vi "Print.vi"(8 "error in":errorcluster, 11 "Object Type Base in":refnum<class "Object Type Base.lvclass">) -> (0 "error out":errorcluster, 2 "Fields":map{string, string}(c390), 3 "Object Type Base out":refnum<class "Object Type Base.lvclass">)   [LabVIEW 2024, in "EDS.lvlib" / "Object Type Base.lvclass"]
uses:
  Object Type Base.lvclass
  Object Type.ctl
  Data Type.ctl
  Access Type.ctl
  Object Type Base.lvclass/Object Type Base.ctl
  EDS.lvlib
panel:
  out "AccessType":T1=enum."const"
  out "DataType":T2 items=["BOOLEAN"=1, "INTEGER8"=2, "INTEGER16"=3, "INTEGER32"=4, "UNSIGNED8"=5, "UNSIGNED16"=6, "UNSIGNED32"=7, "REAL32"=8, "VISIBLE_STRING"=9, "OCTET_STRING"=10, "UNICODE_STRING"=11, "TIME_OF_DAY"=12, "TIME_DIFFERENCE"=13, "RESERVED1"=14, "DOMAIN"=15, "INTEGER24"=16, "REAL64"=17, "INTEGER40"=18, "INTEGER48"=19, "INTEGER56"=20, "INTEGER64"=21, "UNSIGNED24"=22, "RESERVED2"=23, "UNSIGNED40"=24, "UNSIGNED48"=25, "UNSIGNED56"=26, "UNSIGNED64"=27, "RESERVED3"=28, "RESERVED4"=29, "RESERVED5"=30, "RESERVED6"=31, "PDO_COMMUNICATION_PARAMETER"=32, "PDO_MAPPING"=33, "SDO_PARAMETER"=34, "IDENTITY"=35, "RESERVED7"=36]
  out "ObjectType":T3 items=["NULL"=0, "DOMAIN"=2, "DEFTYPE"=5, "DEFSTRUCT"=6, "VAR"=7, "ARRAY"=8, "RECORD"=9]
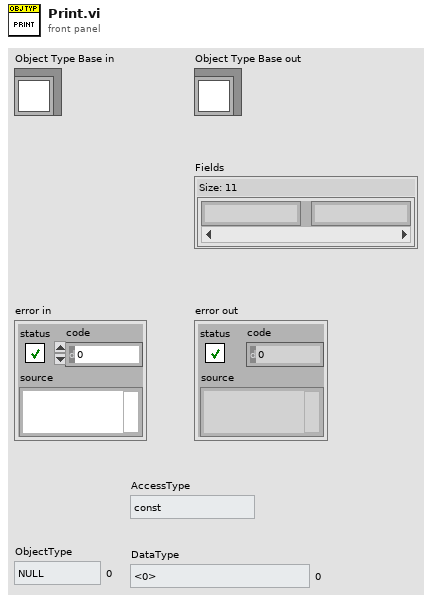
[diagram p1: front panel]
types:
  T1 = typedef "EDS.lvlib/Access Type.ctl" = enum16{"ro", "wo", "rw", "rwr", "rww", "const"}
  T2 = typedef "EDS.lvlib/Data Type.ctl" = u16
  T3 = typedef "EDS.lvlib/Object Type.ctl" = u8
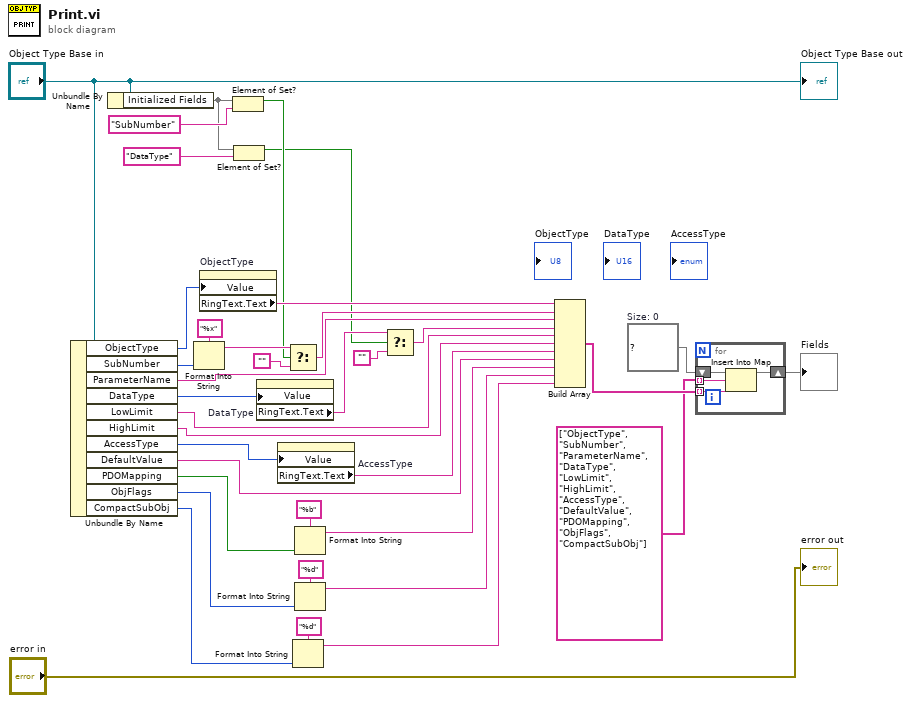
[diagram p0: block diagram]
diagram:
  w30 = map{string, string} {}  # Size: 0
  n1 = Unbundle By Name("Object Type Base in") -> ("ObjectType"=w37:T3, "SubNumber"=w36:u8, "ParameterName"=w27:string, "DataType"=w34:T2, "LowLimit"=w25:string, "HighLimit"=w24:string, "AccessType"=w33:T1, "DefaultValue"=w22:string, "PDOMapping"=w20:bool, "ObjFlags"=w31:u32, "CompactSubObj"=w16:u8)
  n2 = Unbundle By Name("Object Type Base in") -> ("Initialized Fields"=w5:set{string})
  n3 = Format Into String(format string="%x", w36) -> (resulting string=w28:string)  [unwired: 2 in, 1 out]
  n4 = property on="ObjectType" class="Ring (strict)"("Value"=w37) -> ("RingText.Text"=w29:string)  [unwired: 2 in, 2 out]
  n5 = Element of Set?(10:"SubNumber" ("element"), 11:w5) -> (3:w7:bool)
  n6 = Element of Set?(10:"DataType" ("element"), 11:w5) -> (3:w2:bool)
  n7 = property on="DataType" class="Ring (strict)"("Value"=w34) -> ("RingText.Text"=w26:string)  [unwired: 2 in, 2 out]
  n8 = property on="AccessType" class="Enum (strict)"("Value"=w33) -> ("RingText.Text"=w23:string)  [unwired: 2 in, 2 out]
  n9 = Select(t=w28, s=w7, f="") -> (s? t:f=w8:string)
  n10 = Format Into String(format string="%d", w16) -> (resulting string=w15:string)  [unwired: 2 in, 1 out]
  n11 = Format Into String(format string="%b", w20) -> (resulting string=w19:string)  [unwired: 2 in, 1 out]
  n12 = Format Into String(format string="%d", w31) -> (resulting string=w18:string)  [unwired: 2 in, 1 out]
  n13 = Select(t=w26, s=w2, f="") -> (s? t:f=w3:string)
  n14 = Build Array(w29, w8, w27, w3, w25, w24, w23, w22, w19, w18, w15) -> (w14:string[])
  n15 = for {
    shift-right: [w40] -> w13
    shift-left: w30 -> [w41]
    tunnel: string[] ["ObjectType", "SubNumber", "ParameterName", "DataType", "LowLimit", "HighLimit", "AccessType", "DefaultValue", "PDOMapping", "ObjFlags", "CompactSubObj"] -> [w39] mode=indexing
    tunnel: w14 -> [w38] mode=indexing
    n16 = Insert Into Map(map in=w41, key=w39, value=w38) -> (map out=w40:map{string, string})  [unwired: 2 out]
  }
  "Fields" <- w13
  "error out" <- "error in"
  "Object Type Base out" <- "Object Type Base in"
